vi "config.Read.vi"(8 "error in":errorcluster, 11 "camera.nit in":refnum<class "camera.lvclass">) -> (0 "error out":errorcluster, 2 "data value":T1)   [LabVIEW 2020, in "camera.lvclass"]
uses:
  camera.lvclass
  _controls/config.ctl
  camera.lvclass/camera.ctl
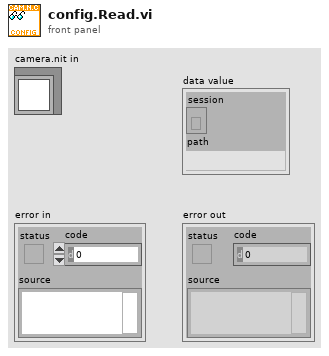
[diagram p1: front panel]
types:
  T1 = typedef "camera.lvclass/config.ctl" = cluster{"session":refnum<k35>, "path":path}
  T2 = typedef "camera.nit.lvclass/config.ctl" = cluster{"session":refnum<k35>, "path":path}
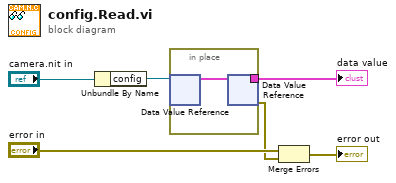
[diagram p0: block diagram]
diagram:
  n1 = Unbundle By Name("camera.nit in") -> ("config"=w4:refnum<data-value>)
  n2 = in-place {
    in-place-border: [w7] -> w1
    n3 = in-place-dvr #1(w4) -> (w7:T2)  [unwired: 1 out]
    n4 = in-place-dvr #1(w7) -> (w2:errorcluster)  [unwired: 1 out]
  }
  "data value" <- w1
  n5 = Merge Errors("error in", w2) -> (→"error out":errorcluster)
